vi "MainProgram.vi"() -> ()   [LabVIEW 2011]
uses:
  CP que.ctl
  Global PhaseStandalone.vi
  JTrkAPI.llb/TrackerDLL.vi
  <vilib>/Utility/file.llb/Write To Spreadsheet File (string).vi
  <vilib>/Utility/file.llb/Read From Spreadsheet File (string).vi
  <vilib>/Analysis/NI_AALBase.lvlib
panel:
  in  "?":T1(tab)=enum."Zlut"
  in  "Frames":T2={"Start frame"=0, "number of frames"=25, "display frame "=0, "track every nd frame "=1, "Track all frames"=TRUE, "active frame"=0}
  out "image size 2":i32[](array[numeric])
  in  "Tracking":T3={"RminZ (pix)"=5, "Rmax (pix)"=25, "angular pixel \ncoverage factor"=0.7, "radial pixel \ncoverage factor"=3.0}
  in  "Calibs":T4={"Zlut number of steps"=200, "um/pix"=0.146, "Z correction factor"=0.88, "Zlut step size (um)"=0.05, "ROI(pix)"=60} {"Zlut step size (um)" format="%_3g"; "Z correction factor" format="%_3g"; "um/pix" format="%_3g"}
  in  "update":bool
  in  "bead number":i32
  in  "Reset all":bool
  in  "Remove bead #":bool
  in  "save beadlist":bool
  in  "load beadlist":bool
  out "# beads":i32
  in  "Beads":cluster{"# ref beads":i32, "overlay":bool}={"# ref beads"=0, "overlay"=TRUE}
  in  "Misc":T5={"save images to new location"=FALSE, "destination"=path "H:/data/images/movies/loop around magnetic bead"}
  in  "autoselect":T6={"select molecules"=FALSE, "exp Lc"=2.4, "restore"=FALSE, "percent"=0.01}
  out "orig time":i32[][](array[numeric])
  out "orig XYZ":dbl[][][](array[numeric])
  out "orig_data.Bead Array":i32[][](array[numeric])
  in  "Tracker DLL (Requires running 32 bit labview)\nPath is relative to application path":path=path "jtrk-labview.dll"
  in  "files":T7={"LUT path"=path "D:/jkerssemakers/My Documents/MB_Data/MB_Labview_Test_Data/40x images Marijn/tmp_133", "Trace path"=path "D:/jkerssemakers/My Documents/MB_Data/MB_Labview_Test_Data/40x images Marijn/tmp_161", " folders #"=1, "base path"=path "D:/jcnossen1/2012-11-23", "use trace"=FALSE, "use base"=TRUE, "LUT tmp"=4, "Trace tmp"=11, "active path"=path "D:/jkerssemakers/My Documents/MB_Data/MB_Labview_Test_Data/40x images Marijn/tmp_133"}
  in  "play":bool
  in  "select beads":bool
  in  "Zlut":bool
  in  "track":bool
  in  "do job":bool
  in  "display":bool
  in  "?":enum32{"Display", "Plot", "Zlut", "Job list"}(tab)=enum."Plot"
  in  "Display":cluster{"Go to bead":i32}
  out "?":u8[][](graph)
  in  "plot":T8
  out "X+Y":cluster{"time out":i32[], "xyz um out":dbl[]}[](graph)
  out "Z":cluster{"time out":i32[], "xyz um out":dbl[]}(graph)
  out "Intensity Graph":dbl[][](graph)
  in  "LUT #":i32
  in  "add to job up to":bool
  in  "Trace tmp":i32=14
  in  "load joblist":bool
  in  "save joblist":bool
  in  "delete":bool
  in  "reset":bool
  in  "add to job":bool
  out "Job list":string[][](array[string])
  in  "stop":bool
  # "Trace"
  # "LUT"
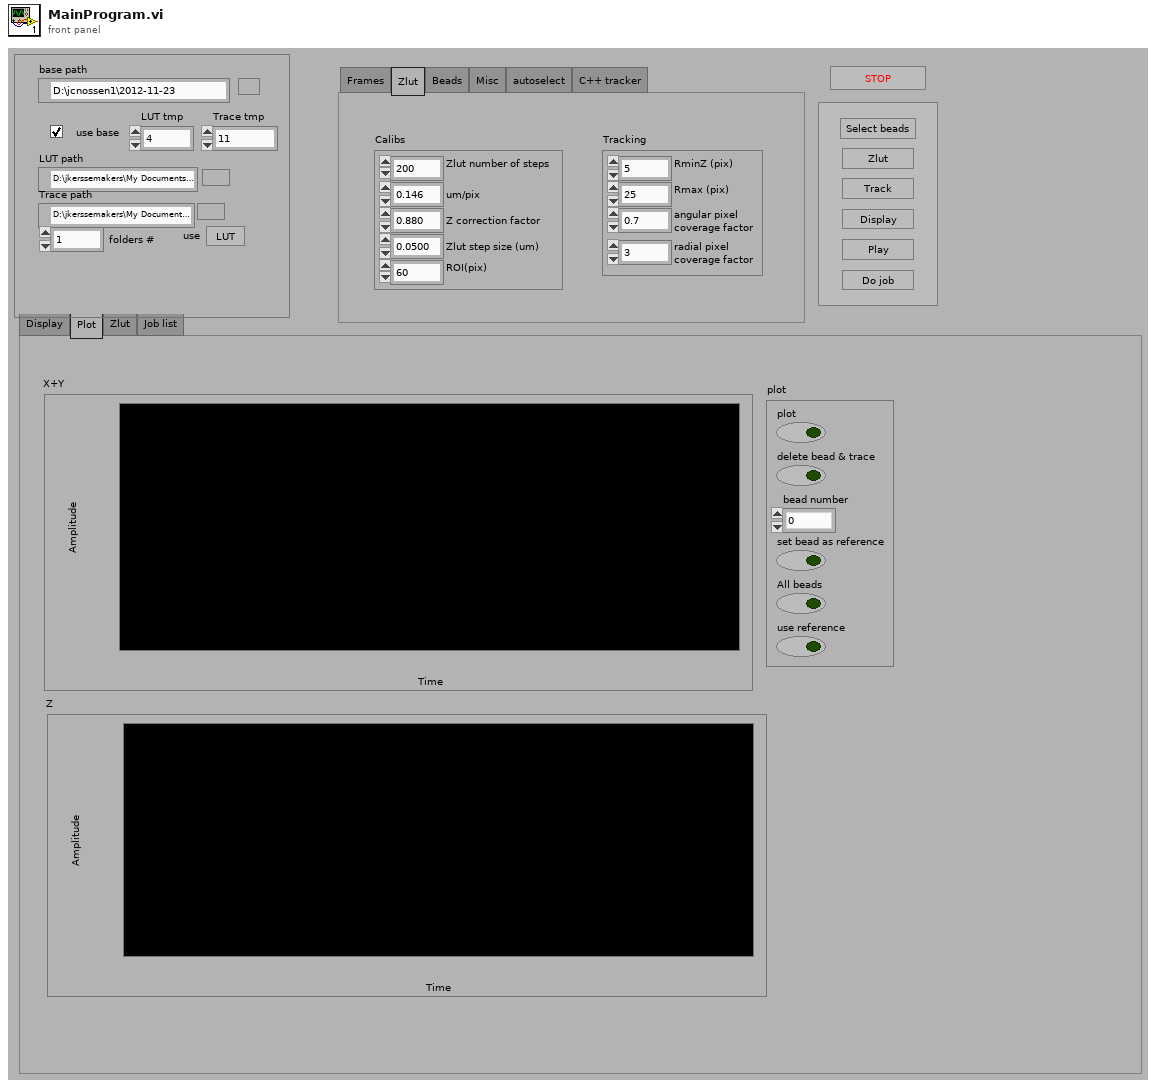
[diagram p1: front panel]
types:
  T1 = enum32{"Frames", "Zlut", "Beads", "Misc", "autoselect", "C++ tracker"}
  T2 = cluster{"Start frame":i32, "number of frames":u32, "display frame ":i32, "track every nd frame ":i32, "Track all frames":bool, "active frame":i32}
  T3 = cluster{"RminZ (pix)":i32, "Rmax (pix)":i32, "angular pixel \ncoverage factor":dbl, "radial pixel \ncoverage factor":dbl}
  T4 = cluster{"Zlut number of steps":i32, "um/pix":dbl, "Z correction factor":dbl, "Zlut step size (um)":dbl, "ROI(pix)":i32}
  T5 = cluster{"save images to new location":bool, "destination":path}
  T6 = cluster{"select molecules":bool, "exp Lc":dbl, "restore":bool, "percent":dbl}
  T7 = cluster{"LUT path":path, "Trace path":path, " folders #":i32, "base path":path, "use trace":bool, "use base":bool, "LUT tmp":i32, "Trace tmp":i32, "active path":path}
  T8 = cluster{"plot":bool, "delete bead & trace":bool, "bead number":i32, "set bead as reference":bool, "All beads":bool, "use reference":bool}
  T9 = typedef "CP que.ctl" = enum16{"idle", "settings", "display", "init", "set beads", "show LUT", "Zlut", "plot", "track", "do job", "joblist", "autoselect", "save", "stop"}
  T10 = enum16{"init", "get", "set single frame", "set all"}
  T11 = typedef "IMAQ Image.ctl" = refnum<image>
  T12 = cluster{"front panel settings":cluster{"files":cluster{"LUT path":path, "Trace path":path, " folders #":i32, "base path":path, "use trace":bool, "use base":bool, "LUT tmp":i32, "Trace tmp":i32, "active path":path}, "Tracking":cluster{"RminZ (pix)":i32, "Rmax (pix)":i32, "angular pixel \ncoverage factor":dbl, "radial pixel \ncoverage factor":dbl}, "Frames":cluster{"Start frame":i32, "number of frames":u32, "display frame ":i32, "track every nd frame ":i32, "Track all frames":bool, "active frame":i32}, "Calibs":cluster{"Zlut number of steps":i32, "pix/um":dbl, "Z correction factor":dbl, "Zlut step size (um)":dbl, "ROI(pix)":i32}, "Beads":cluster{"number of ref beads":i32, "overlay":bool}, "Misc":cluster{"save images to new location":bool, "destination":path}}, "data":cluster{"Image":T11, "image size":i32[], "Bead Array":i32[][], "overlay image":T11, "# beads":i32, "Job list":string[][], "job running":bool, "job #":i32, "folders to go":i32}}
  T13 = cluster{"files":cluster{"LUT path":path, "Trace path":path, " folders #":i32, "base path":path, "use trace":bool, "use base":bool, "LUT tmp":i32, "Trace tmp":i32, "active path":path}, "Tracking":cluster{"RminZ (pix)":i32, "Rmax (pix)":i32, "angular pixel \ncoverage factor":dbl, "radial pixel \ncoverage factor":dbl}, "Frames":cluster{"Start frame":i32, "number of frames":u32, "display frame ":i32, "track every nd frame ":i32, "Track all frames":bool, "active frame":i32}, "Calibs":cluster{"Zlut number of steps":i32, "um/pix":dbl, "Z correction factor":dbl, "Zlut step size (um)":dbl, "ROI(pix)":i32}, "Beads":cluster{"# ref beads":i32, "overlay":bool}, "Misc":cluster{"save images to new location":bool, "destination":path}}
  T14 = cluster{"ROI1":i32, "Rmax (pix)":i32, "RminZ (pix)":i32, "LUTs":dbl[][][], "use trace":bool, "angular pixel\n coverage factor":dbl, "radial pixel\n coverage factor":dbl}
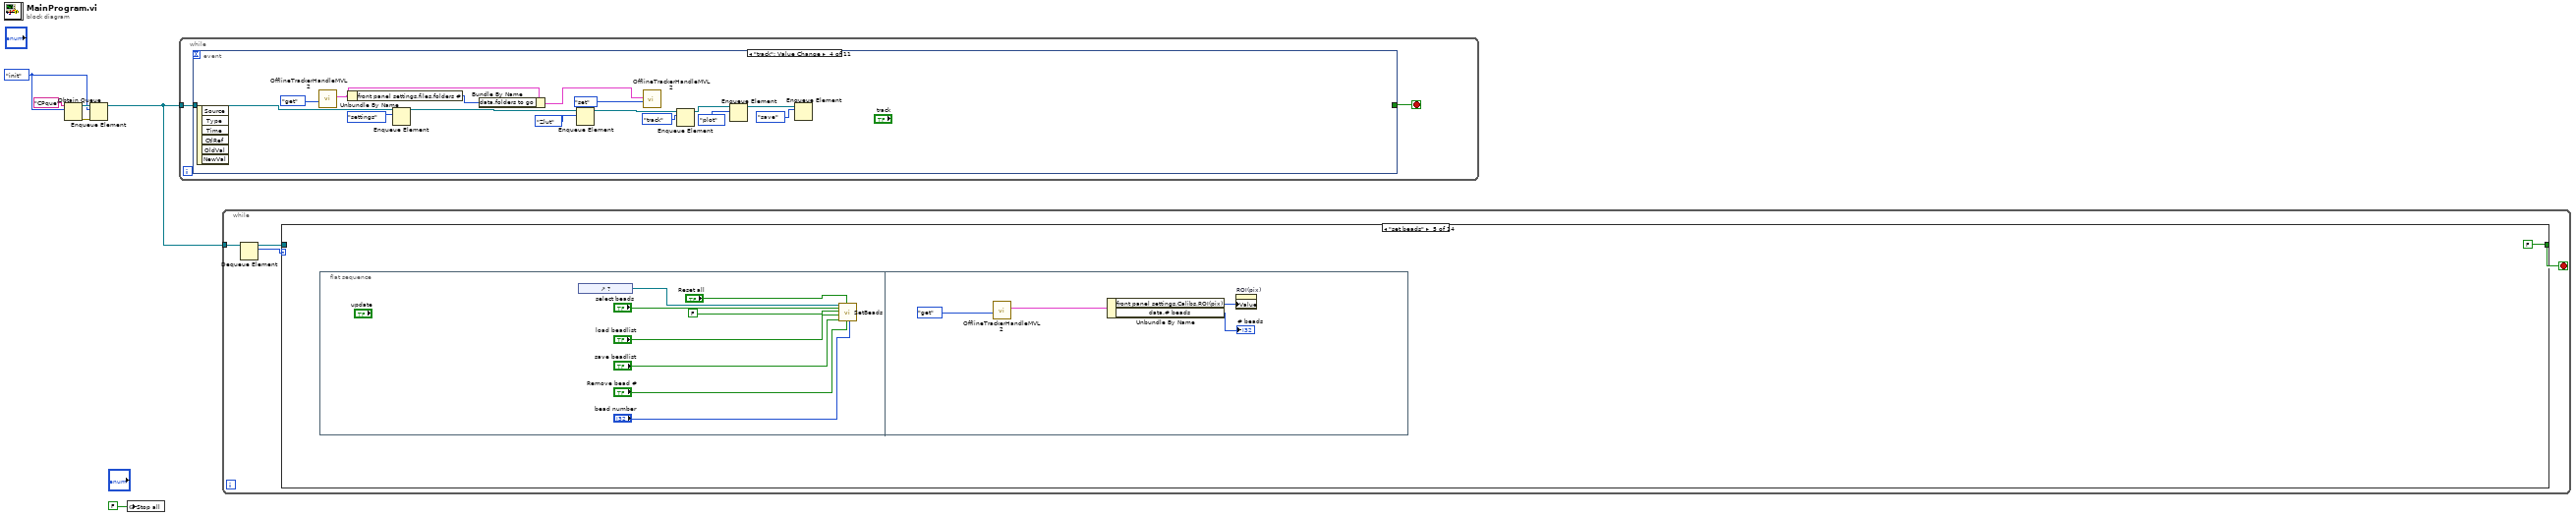
[diagram p0: block diagram]
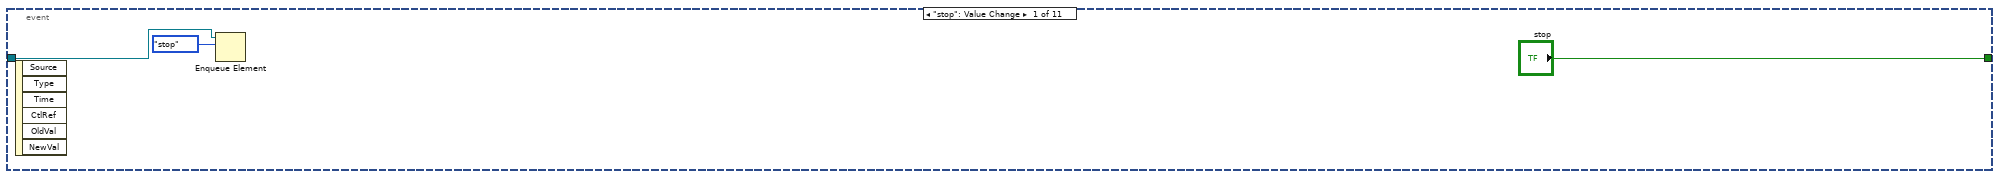
[diagram p2: hidden frame]
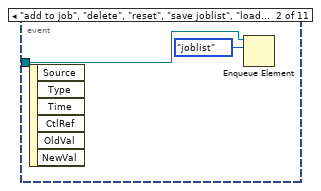
[diagram p3: hidden frame]
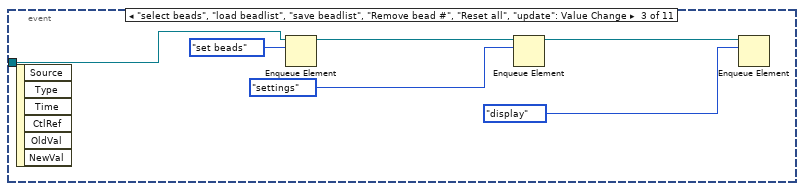
[diagram p4: hidden frame]
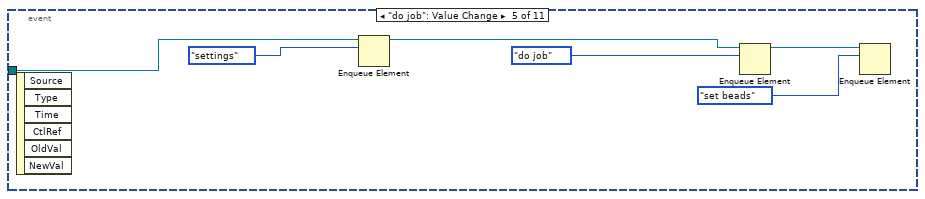
[diagram p5: hidden frame]
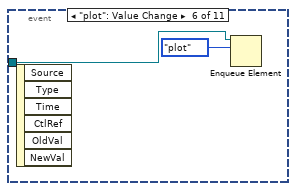
[diagram p6: hidden frame]
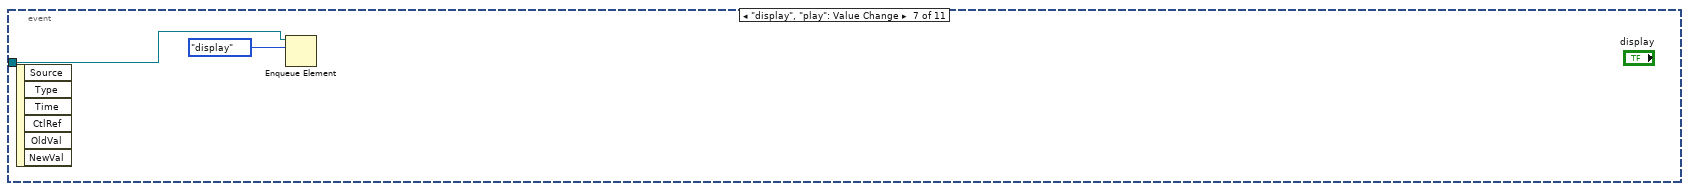
[diagram p7: hidden frame]
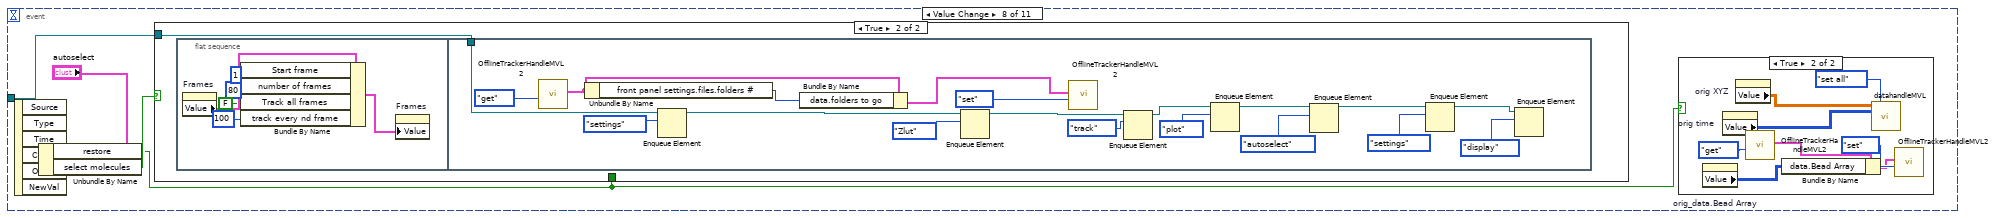
[diagram p8: hidden frame]
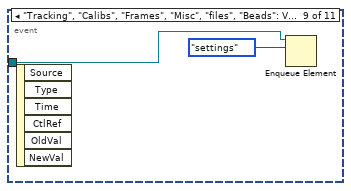
[diagram p11: hidden frame]
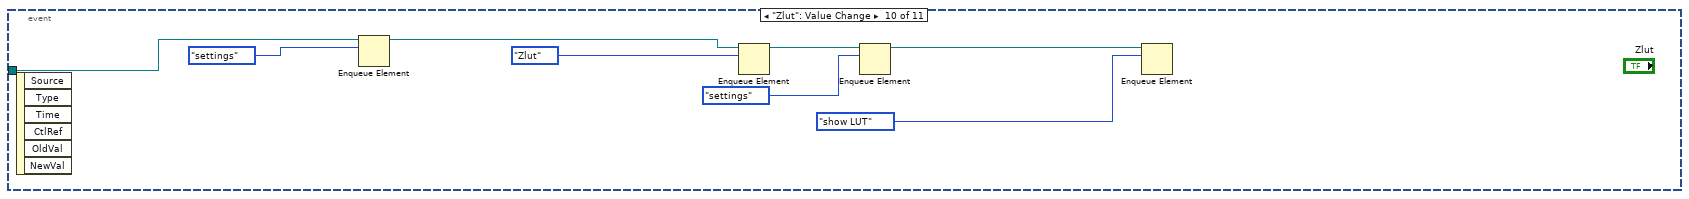
[diagram p12: hidden frame]
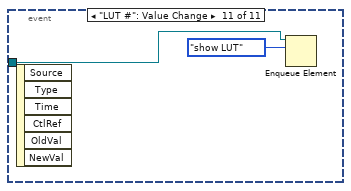
[diagram p13: hidden frame]
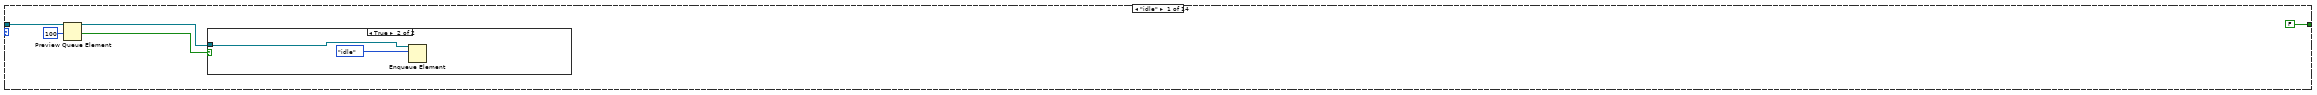
[diagram p14: hidden frame]
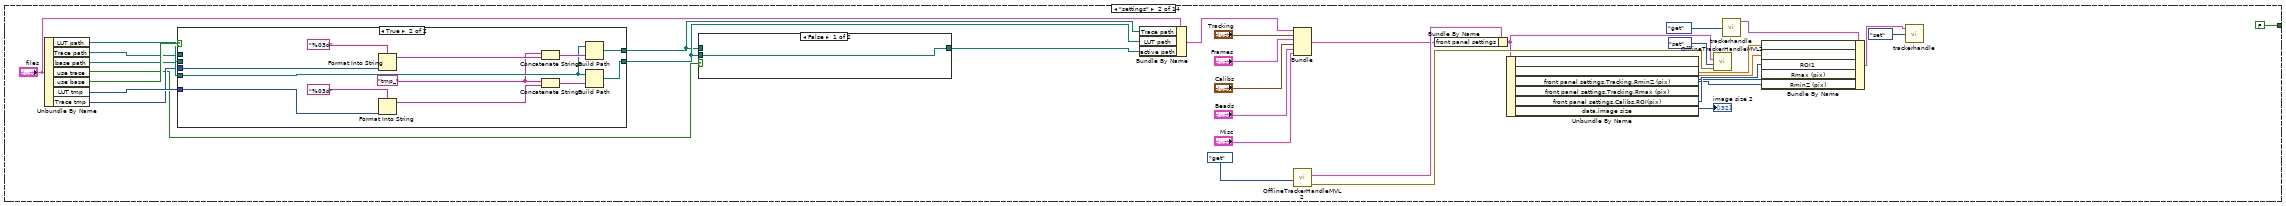
[diagram p16: hidden frame]
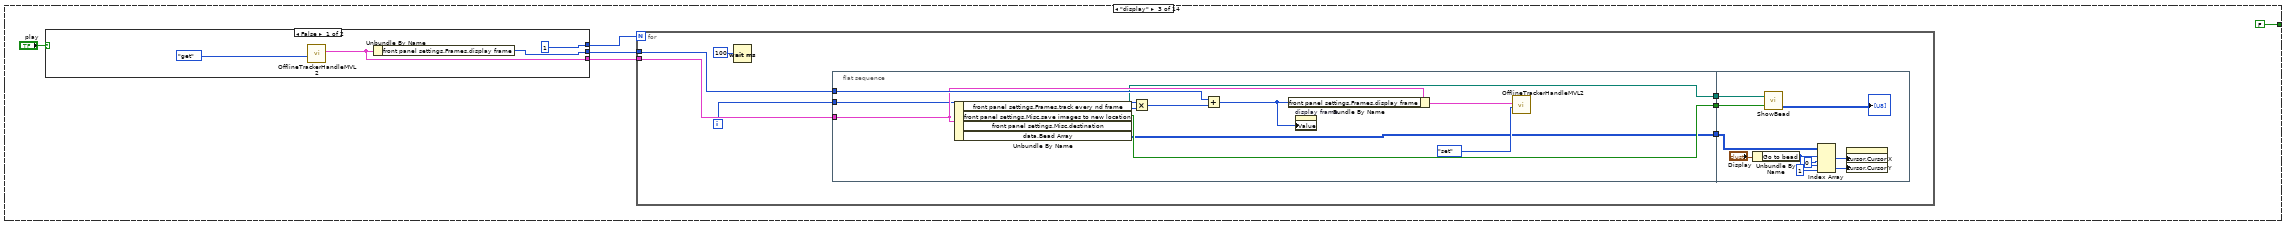
[diagram p19: hidden frame]
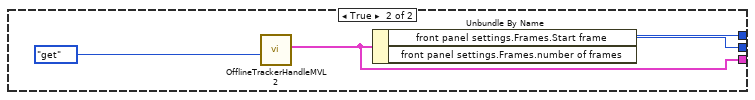
[diagram p20: hidden frame]
diagram:
  w3 = CP_que."init" ("CP que")
  n1 = Obtain Queue(name (unnamed)="CPque", element data type=w3) -> (queue out=w5:refnum<queue>, error out=w4:errorcluster)  [unwired: 3 in, 1 out]
  n2 = Enqueue Element(queue=w5, element=w3, error in (no error)=w4) -> (queue out=w2:refnum<queue>)  [unwired: 3 out]
  n3 = global write "Global PhaseStandalone.vi" "Stop all"(FALSE ("stop")) -> ()
  n4 = while {
    tunnel: w2 -> [w8]
    stop <- w7 stop-if-true
    n5 = event shown="[3] \"track\": Value Change" {
      selector: _ -> [_ _ _ _ _ _ _ _ _ _ _]
      dyn-events: _ -> [_ _ _ _ _ _ _ _ _ _ _]
      timeout: _ -> [_ _ _ _ _ _ _ _ _ _ _]
      tunnel: w8 -> [w11 w13 w18 w33 w39 w41 w43 w48 w84 w92 w93]
      tunnel: ["stop" _ _ _ _ _ _ _ _ _ _] -> w7
      event "stop": Value Change {
        n6 = event-data() -> ()  [unwired: 7 out]
        n7 = Enqueue Element(queue=w11, element=CP_que."stop" ("CP que")) -> ()  [unwired: 1 in, 4 out]
      }
      event "add to job", "delete", "reset", "save joblist", "load joblist", "add to job up to": Value Change {
        n8 = event-data() -> ()  [unwired: 7 out]
        n9 = Enqueue Element(queue=w13, element=CP_que."joblist" ("CP que")) -> ()  [unwired: 1 in, 4 out]
      }
      event "select beads", "load beadlist", "save beadlist", "Remove bead #", "Reset all", "update": Value Change {
        n10 = event-data() -> ()  [unwired: 7 out]
        n11 = Enqueue Element(queue=w18, element=CP_que."set beads" ("CP que")) -> (queue out=w16:refnum<queue>)  [unwired: 1 in, 3 out]
        n12 = Enqueue Element(queue=w16, element=CP_que."settings" ("CP que")) -> (queue out=w14:refnum<queue>)  [unwired: 1 in, 3 out]
        n13 = Enqueue Element(queue=w14, element=CP_que."display" ("CP que")) -> ()  [unwired: 1 in, 4 out]
      }
      event "track": Value Change {
        n14 = event-data() -> ()  [unwired: 7 out]
        n15 = call "OfflineTrackerHandleMVL2.vi"("action"=enum16{"get", "set"}."get") -> ("out"=w22:T12)  [unwired: 5 in, 1 out]
        n16 = Unbundle By Name(w22) -> ("front panel settings.files.folders #"=w20:i32)
        n17 = Enqueue Element(queue=w33, element=CP_que."settings" ("CP que")) -> (queue out=w32:refnum<queue>)  [unwired: 1 in, 3 out]
        n18 = Bundle By Name(cluster=w22, "data.folders to go"=w20) -> (w21:T12)
        n19 = Enqueue Element(queue=w32, element=CP_que."Zlut" ("CP que")) -> (queue out=w25:refnum<queue>)  [unwired: 1 in, 3 out]
        n20 = call "OfflineTrackerHandleMVL2.vi"("action"=enum16{"get", "set"}."set", "in"=w21) -> ()  [unwired: 4 in, 2 out]
        n21 = Enqueue Element(queue=w25, element=CP_que."track" ("CP que")) -> (queue out=w28:refnum<queue>)  [unwired: 1 in, 3 out]
        n22 = Enqueue Element(queue=w28, element=CP_que."plot" ("CP que")) -> (queue out=w26:refnum<queue>)  [unwired: 1 in, 3 out]
        n23 = Enqueue Element(queue=w26, element=CP_que."save" ("CP que")) -> ()  [unwired: 1 in, 4 out]
      }
      event "do job": Value Change {
        n24 = event-data() -> ()  [unwired: 7 out]
        n25 = Enqueue Element(queue=w39, element=CP_que."settings" ("CP que")) -> (queue out=w37:refnum<queue>)  [unwired: 1 in, 3 out]
        n26 = Enqueue Element(queue=w37, element=CP_que."do job" ("CP que")) -> (queue out=w35:refnum<queue>)  [unwired: 1 in, 3 out]
        n27 = Enqueue Element(queue=w35, element=CP_que."set beads" ("CP que")) -> ()  [unwired: 1 in, 4 out]
      }
      event "plot": Value Change {
        n28 = event-data() -> ()  [unwired: 7 out]
        n29 = Enqueue Element(queue=w41, element=CP_que."plot" ("CP que")) -> ()  [unwired: 1 in, 4 out]
      }
      event "display", "play", "Display.Go to bead": Value Change {
        n30 = event-data() -> ()  [unwired: 7 out]
        n31 = Enqueue Element(queue=w43, element=CP_que."display" ("CP que")) -> ()  [unwired: 1 in, 4 out]
      }
      event "autoselect.select molecules", "autoselect.restore": Value Change {
        n32 = event-data() -> ()  [unwired: 7 out]
        n33 = Unbundle By Name("autoselect") -> ("restore"=w45:bool, "select molecules"=w46:bool)
        n34 = case shown="True" w46 {
          tunnel: w48 -> [_ w49]
          tunnel: w45 -> [_ _]
          frame False {
          }
          frame True {
            n35 = flat-sequence {
              tunnel: w49 -> [w69]
              frame #0 {
                n36 = property on="Frames" class="Clust (strict)"() -> ("Value"=w55:T2)  [unwired: 2 in, 2 out]
                n37 = Bundle By Name(cluster=w55, "Start frame"=1, "number of frames"=u32 80, "Track all frames"=FALSE, "track every nd frame"=100) -> (w54:T2)
                n38 = property on="Frames" class="Clust (strict)"("Value"=w54) -> ()  [unwired: 2 in, 2 out]
              }
              frame #1 {
                n39 = call "OfflineTrackerHandleMVL2.vi"("action"=enum16{"get", "set"}."get") -> ("out"=w59:T12)  [unwired: 5 in, 1 out]
                n40 = Unbundle By Name(w59) -> ("front panel settings.files.folders #"=w57:i32)
                n41 = Enqueue Element(queue=w69, element=CP_que."settings" ("CP que")) -> (queue out=w67:refnum<queue>)  [unwired: 1 in, 3 out]
                n42 = Bundle By Name(cluster=w59, "data.folders to go"=w57) -> (w58:T12)
                n43 = Enqueue Element(queue=w67, element=CP_que."Zlut" ("CP que")) -> (queue out=w62:refnum<queue>)  [unwired: 1 in, 3 out]
                n44 = call "OfflineTrackerHandleMVL2.vi"("action"=enum16{"get", "set"}."set", "in"=w58) -> ()  [unwired: 4 in, 2 out]
                n45 = Enqueue Element(queue=w62, element=CP_que."track" ("CP que")) -> (queue out=w63:refnum<queue>)  [unwired: 1 in, 3 out]
                n46 = Enqueue Element(queue=w63, element=CP_que."plot" ("CP que")) -> (queue out=w56:refnum<queue>)  [unwired: 1 in, 3 out]
                n47 = Enqueue Element(queue=w56, element=CP_que."autoselect" ("CP que")) -> (queue out=w72:refnum<queue>)  [unwired: 1 in, 3 out]
                n48 = Enqueue Element(queue=w72, element=CP_que."settings" ("CP que")) -> (queue out=w70:refnum<queue>)  [unwired: 1 in, 3 out]
                n49 = Enqueue Element(queue=w70, element=CP_que."display" ("CP que")) -> ()  [unwired: 1 in, 4 out]
              }
            }
          }
        }
        n50 = case shown="True" w45 {
          frame False {
          }
          frame True {
            n51 = property on="orig_data.Bead Array" class="Arr (strict)"() -> ("Value"=w75:i32[][])  [unwired: 2 in, 2 out]
            n52 = property on="orig time" class="Arr (strict)"() -> ("Value"=w80:i32[][])  [unwired: 2 in, 2 out]
            n53 = property on="orig XYZ" class="Arr (strict)"() -> ("Value"=w81:dbl[][][])  [unwired: 2 in, 2 out]
            n54 = call "OfflineTrackerHandleMVL2.vi"("action"=enum16{"get", "set"}."get") -> ("out"=w77:T12)  [unwired: 5 in, 1 out]
            n55 = Bundle By Name(cluster=w77, "data.Bead Array"=w75) -> (w76:T12)
            n56 = call "datahandleMVL.vi"("xyz array in"=w81, "action"=T10."set all", "Time array in"=w80) -> ()  [unwired: 7 in, 6 out]
            n57 = call "OfflineTrackerHandleMVL2.vi"("action"=enum16{"get", "set"}."set", "in"=w76) -> ()  [unwired: 4 in, 2 out]
          }
        }
      }
      event "Tracking", "Calibs", "Frames", "Misc", "files", "Beads": Value Change {
        n58 = event-data() -> ()  [unwired: 7 out]
        n59 = Enqueue Element(queue=w84, element=CP_que."settings" ("CP que")) -> ()  [unwired: 1 in, 4 out]
      }
      event "Zlut": Value Change {
        n60 = event-data() -> ()  [unwired: 7 out]
        n61 = Enqueue Element(queue=w92, element=CP_que."settings" ("CP que")) -> (queue out=w89:refnum<queue>)  [unwired: 1 in, 3 out]
        n62 = Enqueue Element(queue=w89, element=CP_que."Zlut" ("CP que")) -> (queue out=w87:refnum<queue>)  [unwired: 1 in, 3 out]
        n63 = Enqueue Element(queue=w87, element=CP_que."settings" ("CP que")) -> (queue out=w85:refnum<queue>)  [unwired: 1 in, 3 out]
        n64 = Enqueue Element(queue=w85, element=CP_que."show LUT" ("CP que")) -> ()  [unwired: 1 in, 4 out]
      }
      event "LUT #": Value Change {
        n65 = event-data() -> ()  [unwired: 7 out]
        n66 = Enqueue Element(queue=w93, element=CP_que."show LUT" ("CP que")) -> ()  [unwired: 1 in, 4 out]
      }
    }
  }
  n67 = while {
    tunnel: w2 -> [w98]
    stop <- w95 stop-if-true
    n68 = Dequeue Element(queue=w98) -> (queue out=w97:refnum<queue>, element=w96:T9)  [unwired: 1 in, 3 out]
    n69 = case shown="\"set beads\"" w96 {
      tunnel: w97 -> [w103 _ _ w207 _ _ _ w235 w288 _ w367 _ _ w496]
      tunnel: [FALSE ("Stop all") FALSE ("Stop all") FALSE ("Stop all") FALSE ("Stop all") FALSE ("Stop all") FALSE ("Stop all") FALSE ("stop") FALSE ("Stop all") FALSE ("Stop all") FALSE ("stop") FALSE ("stop") FALSE ("stop") FALSE ("Stop all") w495] -> w95
      frame "idle" {
        n70 = Preview Queue Element(queue=w103, timeout in ms (-1)=100) -> (queue out=w100:refnum<queue>, timed out?=w101:bool)  [unwired: 1 in, 2 out]
        n71 = case shown="True" w101 {
          tunnel: w100 -> [_ w105]
          frame False {
          }
          frame True {
            n72 = Enqueue Element(queue=w105, element=CP_que."idle" ("CP que")) -> ()  [unwired: 1 in, 4 out]
          }
        }
      }
      frame "settings" {
        n73 = Unbundle By Name("files") -> ("LUT path"=w127:path, "Trace path"=w126:path, "base path"=w130:path, "use trace"=w125:bool, "use base"=w131:bool, "LUT tmp"=w129:i32, "Trace tmp"=w128:i32)
        n74 = case shown="True" w131 {
          tunnel: w130 -> [_ w148]
          tunnel: w129 -> [_ w146]
          tunnel: w128 -> [_ w145]
          tunnel: w127 -> [w143 _]
          tunnel: w126 -> [w142 _]
          tunnel: [w142 w152] -> w122
          tunnel: [w143 w147] -> w123
          frame False {
          }
          frame True {
            w144 = "tmp_" ("string")
            n75 = Format Into String(format string="%03d", w145) -> (resulting string=w154:string)  [unwired: 2 in, 1 out]
            n76 = Format Into String(format string="%03d", w146) -> (resulting string=w150:string)  [unwired: 2 in, 1 out]
            n77 = Concatenate Strings(w144, w154) -> (w153:string)
            n78 = Concatenate Strings(w144, w150) -> (w149:string)
            n79 = Build Path(base path=w148, name or relative path=w153) -> (appended path=w152:path)
            n80 = Build Path(base path=w148, name or relative path=w149) -> (appended path=w147:path)
          }
        }
        n81 = case shown="False" w125 {
          tunnel: w122 -> [_ w141]
          tunnel: [w140 w141] -> w120
          tunnel: w123 -> [w140 _]
          frame False {
          }
          frame True {
          }
        }
        n82 = Bundle By Name(cluster="files", "Trace path"=w122, "LUT path"=w123, "active path"=w120) -> (w121:T7)
        n83 = Bundle("files"=w121, "Tracking"="Tracking", "Frames"="Frames", "Calibs"="Calibs", "Beads"="Beads", "Misc"="Misc") -> (w117:T13)  [unwired: 1 in]
        n84 = call "OfflineTrackerHandleMVL2.vi"("action"=enum16{"get", "set"}."get") -> ("error out"=w132:errorcluster, "out"=w118:T12)  [unwired: 5 in]
        n85 = Bundle By Name(cluster=w118, "front panel settings"=w117) -> (w115:T12)
        n86 = Unbundle By Name(w115) -> ("front panel settings.Tracking.angular pixel \ncoverage factor"=w107:dbl, "front panel settings.Tracking.radial pixel \ncoverage factor"=w106:dbl, "front panel settings.Tracking.RminZ (pix)"=w108:i32, "front panel settings.Tracking.Rmax (pix)"=w109:i32, "front panel settings.Calibs.ROI(pix)"=w110:i32, "data.image size"=→"image size 2":i32[])
        n87 = call "OfflineTrackerHandleMVL2.vi"("error in"=w132, "action"=enum16{"get", "set"}."set", "in"=w115) -> ()  [unwired: 3 in, 2 out]
        n88 = call "trackerhandle.vi"("action"=enum16{"get", "set"}."get") -> ("output Cluster"=w112:T14)  [unwired: 2 in, 2 out]
        n89 = Bundle By Name(cluster=w112, "angular pixel\n coverage factor"=w107, "radial pixel\n coverage factor"=w106, "ROI1"=w110, "Rmax (pix)"=w109, "RminZ (pix)"=w108) -> (w111:T14)
        n90 = call "trackerhandle.vi"("action"=enum16{"get", "set"}."set", "input Cluster"=w111) -> ()  [unwired: 1 in, 3 out]
      }
      frame "display" {
        n91 = case shown="False" "play" {
          tunnel: [u32 1 ("number of frames") w167] -> w159
          tunnel: [w161 w166] -> w158
          tunnel: [w162 w165] -> w157
          frame False {
            n92 = call "OfflineTrackerHandleMVL2.vi"("action"=enum16{"get", "set"}."get") -> ("out"=w162:T12)  [unwired: 5 in, 1 out]
            n93 = Unbundle By Name(w162) -> ("front panel settings.Frames.display frame"=w161:i32)
          }
          frame True {
            n94 = call "OfflineTrackerHandleMVL2.vi"("action"=enum16{"get", "set"}."get") -> ("out"=w165:T12)  [unwired: 5 in, 1 out]
            n95 = Unbundle By Name(w165) -> ("front panel settings.Frames.Start frame"=w166:i32, "front panel settings.Frames.number of frames"=w167:u32)
          }
        }
        n96 = for {
          N: w159 -> [_]
          tunnel: w158 -> [w174]
          tunnel: w157 -> [w173]
          i -> [w172]
          n97 = Wait (ms)(milliseconds to wait=u32 100) -> ()  [unwired: 1 out]
          n98 = flat-sequence {
            tunnel: w174 -> [w186]
            tunnel: w173 -> [w183]
            tunnel: w172 -> [w181]
            tunnel: [w178] -> w171
            tunnel: [w177] -> w170
            tunnel: [w176] -> w169
            tunnel: w171 -> [w195]
            tunnel: w170 -> [w194]
            tunnel: w169 -> [w192]
            frame #0 {
              n99 = Unbundle By Name(w183) -> ("front panel settings.Frames.track every nd frame"=w182:i32, "front panel settings.Misc.save images to new location"=w177:bool, "front panel settings.Misc.destination"=w178:path, "data.Bead Array"=w176:i32[][])
              n100 = Multiply(x=w181, y=w182) -> (x*y=w180:i32)
              n101 = Add(x=w186, y=w180) -> (x+y=w179:i32)
              n102 = Bundle By Name(cluster=w183, "front panel settings.Frames.display frame"=w179) -> (w184:T12)
              n103 = property on="display frame" class="DigNum (strict)"("Value"=w179) -> ()  [unwired: 2 in, 2 out]
              n104 = call "OfflineTrackerHandleMVL2.vi"("action"=enum16{"get", "set"}."set", "in"=w184) -> ()  [unwired: 4 in, 2 out]
            }
            frame #1 {
              n105 = Unbundle By Name("Display") -> ("Go to bead"=w190:i32)
              n106 = call "ShowBead.vi"("save images to new location"=w194, "destination"=w195) -> ("ImageplusRois"=→"?":u8[][])  [unwired: 1 out]
              n107 = Index Array(array=w192, index (row) #1=w190, index (col) #1=0 ("disabled index (col)"), index (row) #2=w190, index (col) #2=1 ("disabled index (col)")) -> (element #1=w188:i32, element #2=w187:i32)
              n108 = property class="IntGraph (strict)"("Cursor.Cursor X"=w188, "Cursor.Cursor Y"=w187) -> ()  [unwired: 2 in, 2 out]
            }
          }
        }
      }
      frame "init" {
        n109 = call <vilib>:"Application Directory.vi"() -> ("Application Directory"=w199:path)
        n110 = call "IMAQ Create"("Image Name"="init") -> ("New Image"=w201:T11)  [unwired: 4 in, 1 out]
        n111 = call "OfflineTrackerHandleMVL2.vi"("action"=enum16{"get", "set"}."get") -> ("out"=w203:T12)  [unwired: 5 in, 1 out]
        n112 = Build Path(base path=w199, name or relative path="Tracker DLL (Requires running 32 bit labview)\nPath is relative to application path") -> (appended path=w197:path)
        n113 = Bundle By Name(cluster=w203, "data.overlay image"=w201) -> (w202:T12)
        n114 = global write "TrackerDLL.vi" "tracker DLL path"(w197) -> ()
        n115 = Enqueue Element(queue=w207, element=CP_que."settings") -> ()  [unwired: 1 in, 4 out]
        n116 = call "OfflineTrackerHandleMVL2.vi"("action"=enum16{"get", "set"}."set", "in"=w202) -> ()  [unwired: 4 in, 2 out]
      }
      frame "set beads" {
        n117 = flat-sequence {
          frame #0 {
            n118 = control-ref of="?"() -> (w217:refnum<vi>)
            n119 = call "SetBeads.vi"("IntGraph Refnum"=w217, "Autofind"="select beads", "Add bead"=FALSE, "load beadlist"="load beadlist", "save beadlist"="save beadlist", "Reset all"="Reset all", "Remove bead #"="Remove bead #", "bead number"="bead number") -> ()  [unwired: 1 in, 11 out]
          }
          frame #1 {
            n120 = call "OfflineTrackerHandleMVL2.vi"("action"=enum16{"get", "set"}."get") -> ("out"=w220:T12)  [unwired: 5 in, 1 out]
            n121 = Unbundle By Name(w220) -> ("front panel settings.Calibs.ROI(pix)"=w221:i32, "data.# beads"=→"# beads":i32)
            n122 = property on="ROI(pix)" class="DigNum (strict)"("Value"=w221) -> ()  [unwired: 2 in, 2 out]
          }
        }
      }
      frame "Zlut" {
        n123 = case shown="False" TRUE {
          frame False {
            n124 = case shown="True" FALSE {
              frame False {
              }
              frame True {
                n125 = call "LoadZlut.vi"() -> ()  [unwired: 1 out]
              }
            }
          }
          frame True {
          }
        }
        n126 = call "MakeZlut.vi"() -> ()  [unwired: 1 out]
      }
      frame "show LUT" {
        n127 = call "trackerhandle.vi"("action"=enum16{"get", "set"}."get") -> ("output Cluster"=w228:T14)  [unwired: 2 in, 2 out]
        n128 = Unbundle By Name(w228) -> ("radial pixel\n coverage factor"=w232:dbl, "RminZ (pix)"=w231:i32, "LUTs"=w229:dbl[][][])
        n129 = Reciprocal(x=w232) -> (1/x=w233:dbl)
        n130 = property on="Intensity Graph" class="IntGraph (strict)"("XScale.Multiplier"=w233, "XScale.Offset"=w231) -> ()  [unwired: 2 in, 2 out]
        n131 = Index Array(array=w229, index (dim 0)="LUT #") -> (element=→"Intensity Graph":dbl[][])  [unwired: 2 in]
      }
      frame "track" {
        w242 = TRUE ("front panel settings.files.active path")
        n132 = call "OfflineTrackerHandleMVL2.vi"("action"=enum16{"get", "set"}."get") -> ("out"=w244:T12)  [unwired: 5 in, 1 out]
        n133 = call "trackerhandle.vi"("action"=enum16{"get", "set"}."get") -> ("error out"=w249:errorcluster, "output Cluster"=w250:T14)  [unwired: 2 in, 1 out]
        n134 = Bundle By Name(cluster=w244, "front panel settings.files.use trace"=w242) -> (w243:T12)
        n135 = Bundle By Name(cluster=w250, "use trace"=w242) -> (w248:T14)
        n136 = call "OfflineTrackerHandleMVL2.vi"("action"=enum16{"get", "set"}."set", "in"=w243) -> ()  [unwired: 4 in, 2 out]
        n137 = call "trackerhandle.vi"("error in"=w249, "action"=enum16{"get", "set"}."set", "input Cluster"=w248) -> ("error out"=w247:errorcluster)  [unwired: 2 out]
        n138 = call "Trackit.vi"("error out"=w247) -> ("error out 2"=w240:errorcluster)  [unwired: 10 out]
        n139 = call "OfflineTrackerHandleMVL2.vi"("error in"=w240, "action"=enum16{"get", "set"}."get") -> ("out"=w236:T12)  [unwired: 4 in, 1 out]
        n140 = Unbundle By Name(w236) -> ("data.folders to go"=w239:i32, "front panel settings.files.Trace tmp"=w234:i32)
        n141 = Decrement(x=w239) -> (x-1=w237:i32)
        n142 = Greater Than 0?(x=w237) -> (x > 0?=w238:bool)
        n143 = case shown="True" w238 {
          tunnel: w237 -> [_ w267]
          tunnel: w236 -> [_ w269]
          tunnel: w235 -> [_ w263]
          tunnel: w234 -> [_ w256]
          frame False {
          }
          frame True {
            n144 = Bundle By Name(cluster=w269, "data.folders to go"=w267) -> (w268:T12)
            n145 = Increment(x=w256) -> (x+1=w254:i32)
            n146 = property on="Trace tmp" class="DigNum (strict)"("Value"=w254) -> ()  [unwired: 2 in, 2 out]
            n147 = call "OfflineTrackerHandleMVL2.vi"("action"=enum16{"get", "set"}."set", "in"=w268) -> ("error out"=w255:errorcluster)  [unwired: 4 in, 1 out]
            n148 = Enqueue Element(queue=w263, element=CP_que."settings" ("CP que"), error in (no error)=w255) -> (queue out=w265:refnum<queue>)  [unwired: 3 out]
            n149 = Enqueue Element(queue=w265, element=CP_que."Zlut" ("CP que")) -> (queue out=w261:refnum<queue>)  [unwired: 1 in, 3 out]
            n150 = Enqueue Element(queue=w261, element=CP_que."track" ("CP que")) -> (queue out=w258:refnum<queue>)  [unwired: 1 in, 3 out]
            n151 = Enqueue Element(queue=w258, element=CP_que."plot" ("CP que")) -> (queue out=w257:refnum<queue>)  [unwired: 1 in, 3 out]
            n152 = Enqueue Element(queue=w257, element=CP_que."save" ("CP que")) -> ()  [unwired: 1 in, 4 out]
          }
        }
      }
      frame "plot" {
        w289 = FALSE  # Z only
        n153 = Unbundle By Name("plot") -> ("delete bead & trace"=w275:bool, "bead number"=w277:i32, "set bead as reference"=w278:bool, "All beads"=w276:bool, "use reference"=w274:bool)  [unwired: 1 out]
        n154 = call "Plot_em.vi"("queue out"=w288, "set bead as reference"=w278, "bead number"=w277, "delete bead & trace"=w275, "All beads"=w276, "Z only"=w289, "use reference"=w274) -> ("Array"=w287:cluster{"time out":i32[], "xyz um out":dbl[]}[], "queue out 2"=w271:refnum<queue>)
        n155 = Enqueue Element(queue=w271, element=CP_que."settings" ("CP que")) -> ()  [unwired: 1 in, 4 out]
        n156 = Index Array(array=w287, index #1=0 ("index"), index #2=1 ("index"), index #3=2 ("index")) -> (element #1=w282:cluster{"time out":i32[], "xyz um out":dbl[]}, element #2=w281:cluster{"time out":i32[], "xyz um out":dbl[]}, element #3=→"Z":cluster{"time out":i32[], "xyz um out":dbl[]})
        n157 = Build Array(w282, w281) -> (→"X+Y":cluster{"time out":i32[], "xyz um out":dbl[]}[])
      }
      frame "joblist" {
        n158 = call "OfflineTrackerHandleMVL2.vi"("action"=enum16{"get", "set"}."get") -> ("out"=w305:T12)  [unwired: 5 in, 1 out]
        n159 = Unbundle By Name(w305) -> ("front panel settings.files.base path"=w299:path, "front panel settings.files.Trace path"=w313:path, "front panel settings.files.LUT path"=w312:path, "data.Job list"=w307:string[][])
        n160 = Path To String(path=w312) -> (string=w309:string)
        n161 = Path To String(path=w313) -> (string=w310:string)
        n162 = Build Path(base path=w299, name or relative path="joblist.txt") -> (appended path=w294:path)
        n163 = Build Array(w309, w310) -> (w290:string[])
        n164 = case shown="True" "add to job" {
          tunnel: w290 -> [_ w365]
          tunnel: w307 -> [w361 w366]
          tunnel: [w361 w364] -> w293
          frame False {
          }
          frame True {
            w362 = FALSE ("save beadlist")
            n165 = Build Array (concatenate)(w366, w365) -> (w364:string[][])
            n166 = call "SetBeads.vi"("Autofind"=w362, "Add bead"=w362, "load beadlist"=w362, "save beadlist"=TRUE, "Reset all"=w362, "Remove bead #"=w362) -> ()  [unwired: 3 in, 11 out]
          }
        }
        n167 = case shown="True" "add to job up to" {
          tunnel: w293 -> [w315 w320]
          tunnel: [w315 w318] -> w292
          tunnel: w290 -> [_ w330]
          frame False {
          }
          frame True {
            n168 = Index Array(array=w330, index #1=0 ("index"), index #2=1 ("index")) -> (element #1=w319:string, element #2=w327:string)
            n169 = String To Path(string=w327) -> (path=w326:path)
            n170 = Strip Path(path=w326) -> (stripped path=w321:path, name=w325:string)
            n171 = Decimal String To Number(string=w325, offset=4) -> (number=w322:i32)  [unwired: 1 in, 1 out]
            n172 = Subtract(x="Trace tmp", y=w322) -> (x-y=w317:i32)
            n173 = Increment(x=w317) -> (x+1=w316:i32)
            n174 = for {
              N: w316 -> [_]
              tunnel: w322 -> [w344]
              tunnel: w321 -> [w337]
              tunnel: w319 -> [w335]
              shift-right: [w331] -> w318
              shift-left: w320 -> [w336]
              i -> [w343]
              n175 = Add(x=w344, y=w343) -> (x+y=w341:i32)
              n176 = Format Into String(format string="%03d", w341) -> (resulting string=w339:string)  [unwired: 2 in, 1 out]
              n177 = Concatenate Strings("tmp_" ("string"), w339) -> (w338:string)
              n178 = Build Path(base path=w337, name or relative path=w338) -> (appended path=w334:path)
              n179 = Path To String(path=w334) -> (string=w333:string)
              n180 = Build Array(w335, w333) -> (w332:string[])
              n181 = Build Array (concatenate)(w336, w332) -> (w331:string[][])
            }
          }
        }
        n182 = case shown="False" "reset" {
          tunnel: w292 -> [w359 _]
          tunnel: [w359 string[][] [] ("Job list")] -> w301
          frame False {
          }
          frame True {
          }
        }
        n183 = case shown="True" "delete" {
          tunnel: w301 -> [w351 w356]
          tunnel: [w351 w358] -> w297
          frame False {
          }
          frame True {
            n184 = Array Size(array=w356) -> (size(s)=w355:i32[])
            n185 = Index Array(array=w355, index=0) -> (element=w352:i32)
            n186 = Decrement(x=w352) -> (x-1=w353:i32)
            n187 = Delete From Array(array=w356, length=1, index (row)=w353) -> (array with subset deleted=w358:string[][])  [unwired: 1 in, 1 out]
          }
        }
        n188 = case shown="True" "save joblist" {
          tunnel: w297 -> [_ w350]
          tunnel: w294 -> [_ w349]
          frame False {
          }
          frame True {
            n189 = call-poly <vilib>:"Write To Spreadsheet File.vi"("append to file? (new file:F)"=FALSE, "2D data"=w350, "file path (dialog if empty)"=w349) -> ()  [unwired: 5 in, 1 out]
          }
        }
        n190 = case shown="True" "load joblist" {
          tunnel: w297 -> [w345 _]
          tunnel: [w345 w346] -> w296
          tunnel: w294 -> [_ w347]
          frame False {
          }
          frame True {
            n191 = call-poly <vilib>:"Read From Spreadsheet File.vi"("file path (dialog if empty)"=w347) -> ("all rows"=w346:string[][])  [unwired: 6 in, 4 out]
          }
        }
        "Job list" <- w296
        n192 = Bundle By Name(cluster=w305, "data.Job list"=w296) -> (w304:T12)
        n193 = call "OfflineTrackerHandleMVL2.vi"("action"=enum16{"get", "set"}."set", "in"=w304) -> ()  [unwired: 4 in, 2 out]
      }
      frame "do job" {
        n194 = stacked-sequence {
          tunnel: w367 -> [_ _ w399 w406]
          frame #0 {
            n195 = disable-structure shown="Disabled" {
              frame Disabled {
                n196 = property on="Track all frames" class="Bool (strict)"("Value"=TRUE) -> ()  [unwired: 2 in, 2 out]
                n197 = property on="Start frame" class="DigNum (strict)"("Value"=0) -> ()  [unwired: 2 in, 2 out]
                n198 = property on="track every nd frame" class="DigNum (strict)"("Value"=1) -> ()  [unwired: 2 in, 2 out]
              }
              frame Enabled {
              }
            }
            n199 = call "OfflineTrackerHandleMVL2.vi"("action"=enum16{"get", "set"}."get") -> ("out"=w376:T12)  [unwired: 5 in, 1 out]
            n200 = Unbundle By Name(w376) -> ("data.Job list"=w370:string[][], "data.job #"=w374:i32)
            n201 = property on="use base" class="Bool (strict)"("Value"=FALSE) -> ()  [unwired: 2 in, 2 out]
            n202 = case shown="True" "do job" {
              selector: "do job" -> [_ w390]
              tunnel: w376 -> [w389 w393]
              tunnel: [w389 w392] -> w375
              tunnel: w374 -> [w388 _]
              tunnel: [w388 w391] -> w373
              frame False {
              }
              frame True {
                w391 = 0 ("data.job #")
                n203 = Bundle By Name(cluster=w393, "data.job running"=w390, "data.job #"=w391) -> (w392:T12)
              }
            }
            n204 = Index Array(array=w370, index (row) #1=w373, index (col) #1=0 ("index"), index (row) #2=w373, index (col) #2=1 ("index")) -> (element #1=w381:string, element #2=w380:string)
            n205 = String To Path(string=w381) -> (path=w372:path)
            n206 = String To Path(string=w380) -> (path=w371:path)
            n207 = property on="LUT path" class="Path"("Value"=w372) -> ()  [unwired: 2 in, 2 out]
            n208 = property on="Trace path" class="Path"("Value"=w371) -> ()  [unwired: 2 in, 2 out]
            n209 = Bundle By Name(cluster=w375, "front panel settings.files.LUT path"=w372, "front panel settings.files.Trace path"=w371) -> (w382:T12)
            n210 = call "OfflineTrackerHandleMVL2.vi"("action"=enum16{"get", "set"}."set", "in"=w382) -> ()  [unwired: 4 in, 2 out]
          }
          frame #1 {
            w395 = FALSE ("save beadlist")
            n211 = call "SetBeads.vi"("Autofind"=w395, "Add bead"=w395, "load beadlist"=TRUE, "save beadlist"=w395, "Reset all"=w395, "Remove bead #"=w395) -> ()  [unwired: 3 in, 11 out]
          }
          frame #2 {
            n212 = Enqueue Element(queue=w399, element=CP_que."settings" ("CP que")) -> (queue out=w404:refnum<queue>)  [unwired: 1 in, 3 out]
            n213 = Enqueue Element(queue=w404, element=CP_que."Zlut" ("CP que")) -> (queue out=w396:refnum<queue>)  [unwired: 1 in, 3 out]
            n214 = Enqueue Element(queue=w396, element=CP_que."track" ("CP que")) -> (queue out=w400:refnum<queue>)  [unwired: 1 in, 3 out]
            n215 = Enqueue Element(queue=w400, element=CP_que."plot" ("CP que")) -> (queue out=w397:refnum<queue>)  [unwired: 1 in, 3 out]
            n216 = Enqueue Element(queue=w397, element=CP_que."save" ("CP que")) -> ()  [unwired: 1 in, 4 out]
          }
          frame #3 {
            n217 = call "OfflineTrackerHandleMVL2.vi"("action"=enum16{"get", "set"}."get") -> ("out"=w410:T12)  [unwired: 5 in, 1 out]
            n218 = Unbundle By Name(w410) -> ("data.job #"=w407:i32, "data.Job list"=w414:string[][])
            n219 = Array Size(array=w414) -> (size(s)=w413:i32[])
            n220 = Index Array(array=w413, index=0) -> (element=w409:i32)
            n221 = Decrement(x=w409) -> (x-1=w408:i32)
            n222 = Less?(x=w407, y=w408) -> (x < y?=w411:bool)
            n223 = case shown="True" w411 {
              tunnel: w410 -> [w418 w426]
              tunnel: w407 -> [_ w422]
              tunnel: w406 -> [_ w421]
              frame False {
                n224 = Bundle By Name(cluster=w418, "data.job running"=FALSE) -> (w417:T12)
                n225 = call "OfflineTrackerHandleMVL2.vi"("action"=enum16{"get", "set"}."set", "in"=w417) -> ()  [unwired: 4 in, 2 out]
              }
              frame True {
                n226 = Increment(x=w422) -> (x+1=w423:i32)
                n227 = Enqueue Element(queue=w421, element=CP_que."do job") -> ()  [unwired: 2 in, 3 out]
                n228 = Bundle By Name(cluster=w426, "data.job running"=TRUE, "data.job #"=w423) -> (w425:T12)
                n229 = call "OfflineTrackerHandleMVL2.vi"("action"=enum16{"get", "set"}."set", "in"=w425) -> ()  [unwired: 4 in, 2 out]
              }
            }
          }
        }
      }
      frame "autoselect" {
        n230 = call "datahandleMVL.vi"("action"=T10."get") -> ("XYZ out"=w428:dbl[][][], "time out"=w429:i32[][], "error in 2"=w434:errorcluster)  [unwired: 9 in, 3 out]
        "orig time" <- w429
        "orig XYZ" <- w428
        n231 = call "datahandleMVL.vi"("xyz array in"=dbl[][][] [], "action"=T10."set all", "error in"=w434) -> ("error in 2"=w433:errorcluster)  [unwired: 7 in, 5 out]
        n232 = call "OfflineTrackerHandleMVL2.vi"("action"=enum16{"get", "set"}."get") -> ("out"=w440:T12)  [unwired: 5 in, 1 out]
        n233 = Unbundle By Name(w440) -> ("data.Bead Array"=w442:i32[][])
        "orig_data.Bead Array" <- w442
        n234 = for {
          tunnel: w428 -> [w450]
          tunnel: w442 -> [w464] mode=indexing
          shift-right: [w463] -> w439
          shift-left: i32[][] [] -> [w462]
          shift-right: [w453] -> _
          shift-left: 0 ("length") -> [w454]
          tunnel: w433 -> [_]
          shift-right: [w451] -> w430
          shift-left: w428 -> [w452]
          i -> [w447]
          n235 = call "pix2um&refsubstract.vi"("ref substract"=FALSE, "XYZ in"=w450) -> ("xyz um out"=w449:dbl[][][])  [unwired: 3 out]
          n236 = Index Array(array=w449, index (dim 0) #1=w447, index (dim 2) #1=0 ("disabled index (col)"), index (dim 0) #2=w447, index (dim 2) #2=1 ("disabled index (col)"), index (dim 0) #3=w447, index (dim 2) #3=2 ("disabled index (row)")) -> (element #1=w457:dbl[], element #2=w456:dbl[], element #3=w458:dbl[])  [unwired: 3 in]
          n237 = property on="percent" class="DigNum (strict)"() -> ("Value"=w446:dbl)  [unwired: 2 in, 2 out]
          n238 = Array Subset(array=w458, index=30, length=20) -> (w471:dbl[])
          n239 = Array Subset(array=w458, index=0, length=10) -> (w472:dbl[])
          n240 = property on="exp Lc" class="DigNum (strict)"() -> ("Value"=w467:dbl)  [unwired: 2 in, 2 out]
          n241 = call <vilib>:"Mean.vi"("X"=w472) -> ("mean"=w469:dbl)  [unwired: 1 out]
          n242 = call <vilib>:"Mean.vi"("X"=w471) -> ("mean"=w470:dbl)  [unwired: 1 out]
          n243 = Multiply(x=w446, y=w467) -> (x*y=w466:dbl)
          n244 = Add(x=w470, y=w466) -> (x+y=w468:dbl)
          n245 = Greater?(x=w469, y=w468) -> (0:w465:bool)
          n246 = case shown="True" w465 {
            tunnel: w464 -> [_ w480]
            tunnel: [w477 w479] -> w463
            tunnel: w462 -> [w477 w481]
            tunnel: w458 -> [_ _]
            tunnel: w457 -> [_ _]
            tunnel: w456 -> [_ _]
            tunnel: w454 -> [w476 w485]
            tunnel: [w476 w487] -> w453
            tunnel: w452 -> [w478 w486]
            tunnel: [w478 w482] -> w451
            tunnel: w447 -> [_ w484]
            frame False {
            }
            frame True {
              n247 = Index Array(array=w486, index (dim 0)=w484) -> (element=w483:dbl[][])  [unwired: 2 in]
              n248 = Increment(x=w485) -> (x+1=w487:i32)
              n249 = Build Array (concatenate)(w481, w480) -> (w479:i32[][])
              n250 = Replace Array Subset(array=w486, new element=w483, index (dim 0)=w485) -> (w482:dbl[][][])  [unwired: 2 in]
            }
          }
        }
        n251 = Bundle By Name(cluster=w440, "data.Bead Array"=w439) -> (w438:T12)
        n252 = call "datahandleMVL.vi"("xyz array in"=w430, "action"=T10."set all", "Time array in"=w429) -> ()  [unwired: 7 in, 6 out]
        n253 = call "OfflineTrackerHandleMVL2.vi"("action"=enum16{"get", "set"}."set", "in"=w438) -> ()  [unwired: 4 in, 2 out]
      }
      frame "save" {
        n254 = call "datahandleMVL.vi"("action"=T10."get") -> ("XYZ out"=w491:dbl[][][])  [unwired: 9 in, 5 out]
        n255 = Array Max & Min(array=w491) -> (max value=w490:dbl, min value=w489:dbl)  [unwired: 2 out]
        n256 = Not Equal?(x=w490, y=w489) -> (x != y?=w488:bool)
        n257 = case shown="True" w488 {
          frame False {
          }
          frame True {
            n258 = call "SaveData.vi"() -> ()  [unwired: 2 in, 1 out]
          }
        }
      }
      frame "stop" {
        w495 = TRUE ("stop")
        n259 = Release Queue(queue=w496, force destroy? (F)=TRUE) -> ()  [unwired: 1 in, 3 out]
        n260 = global write "Global PhaseStandalone.vi" "Stop all"(w495) -> ()
      }
    }
  }
